vi "determine warnings.vi"() -> ()   [LabVIEW 2014]
panel:
  out "warning?":bool
  out "warning text":string
  in  "min temp":dbl
  in  "max temp":dbl
  in  "current temp.":dbl
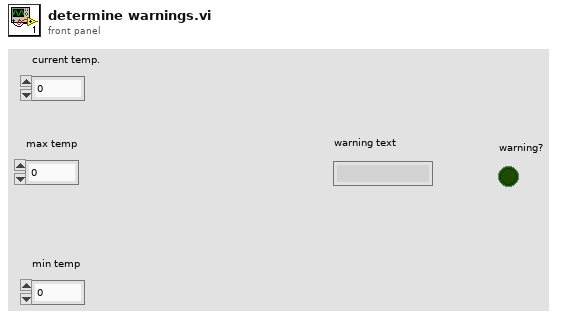
[diagram p1: front panel]
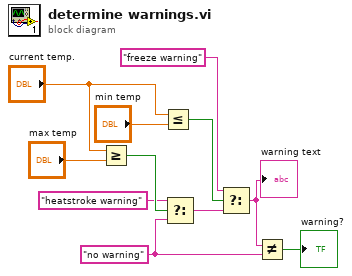
[diagram p0: block diagram]
diagram:
  w2 = "no warning"
  n1 = Greater Or Equal?(x="current temp.", y="max temp") -> (x >= y?=w7:bool)
  n2 = Less Or Equal?(x="current temp.", y="min temp") -> (x <= y?=w8:bool)
  n3 = Select(t="heatstroke warning", s=w7, f=w2) -> (s? t:f=w4:string)
  n4 = Select(t="freeze warning", s=w8, f=w4) -> (s? t:f=w3:string)
  "warning text" <- w3
  n5 = Not Equal?(x=w3, y=w2) -> (x != y?=→"warning?":bool)
